vi "实验4_1.vi"() -> ()   [LabVIEW 2018]
panel:
  out "graph":cluster{i32, i32, dbl[]}[](graph)
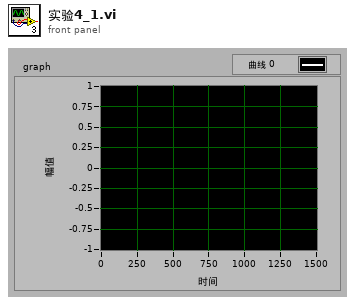
[diagram p1: front panel]
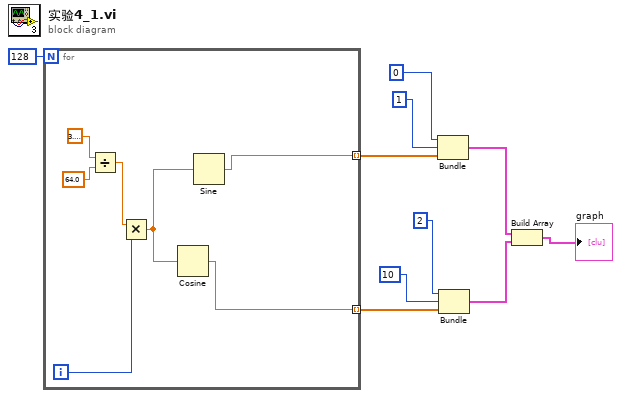
[diagram p0: block diagram]
diagram:
  n1 = for {
    N: 128 -> [_]
    tunnel: [w15] -> w7 mode=indexing
    tunnel: [w14] -> w6 mode=indexing
    i -> [w17]
    n2 = Divide(x=3.141592653589793, y=64.0) -> (x/y=w11:dbl)
    n3 = Multiply(x=w11, y=w17) -> (x*y=w16:dbl)
    n4 = Cosine(x=w16) -> (cos(x)=w14:dbl)
    n5 = Sine(x=w16) -> (sin(x)=w15:dbl)
  }
  n6 = Bundle(0, 1, w7) -> (w3:cluster{i32, i32, dbl[]})  [unwired: 1 in]
  n7 = Bundle(2, 10, w6) -> (w2:cluster{i32, i32, dbl[]})  [unwired: 1 in]
  n8 = Build Array(w3, w2) -> (→"graph":cluster{i32, i32, dbl[]}[])
